vi "Discover Nodes.vi"(8 "error in":errorcluster, 11 "Interactor in":refnum<class "Interactor.lvclass">) -> (0 "error out":errorcluster, 3 "Interactor out":refnum<class "Interactor.lvclass">)   [LabVIEW 2024, in "Interactor.lvlib" / "Interactor.lvclass"]
uses:
  Interactor.lvclass
  Interactor.lvclass/Interactor.ctl
  CANopen Master/CANopen Master.lvclass
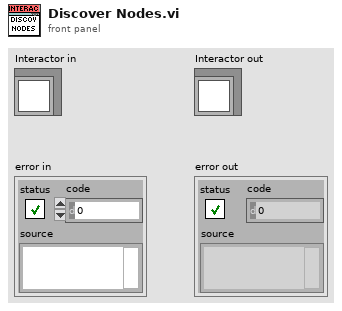
[diagram p1: front panel]
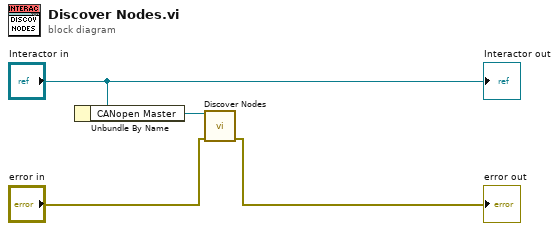
[diagram p0: block diagram]
diagram:
  n1 = Unbundle By Name("Interactor in") -> ("CANopen Master"=w3:refnum<class "CANopen Master.lvclass">)
  n2 = call "Discover Nodes.vi"("error in"="error in", "CANopen Master in"=w3) -> ("error out"=→"error out":errorcluster)  [unwired: 8 in, 1 out]
  "Interactor out" <- "Interactor in"
